vi "Bella_TEA_EnergyMeter_GUI-viremote.vi"() -> (0 "error IO 2":errorcluster)   [LabVIEW 2013]
uses:
  shared programs/GUI_Template/GUI_master/tcp_new_data_event.ctl
  shared programs/GUI_Template/GUI_master/tcp new data cluster.ctl
  VIremote/VIremote.llb/VIremoteFunction.ctl
panel:
  in  "error IO":errorcluster
  in  "Energy Mode::11":enum16{"off", "on"}(ring) caption="Energy Mode"
  in  "triggerlevel::11":dbl=0.5 caption="Trig Level" min=0.0 max=100.0 format="%_4f"
  out "Wavelength::11":i32 caption="Wavelength" min=0 max=5000
  out "tcp data event":T1
  in  "GUIdevice 11":string="BELLA_TEA_PowerMeter"
  in  "insert tag":bool=TRUE
  in  "stop":bool
  out "Reading::11":dbl=0.5 caption="Reading" min=0.0 max=50000.0 format="%_4p"
  # "TEA PLink Energy Meter"
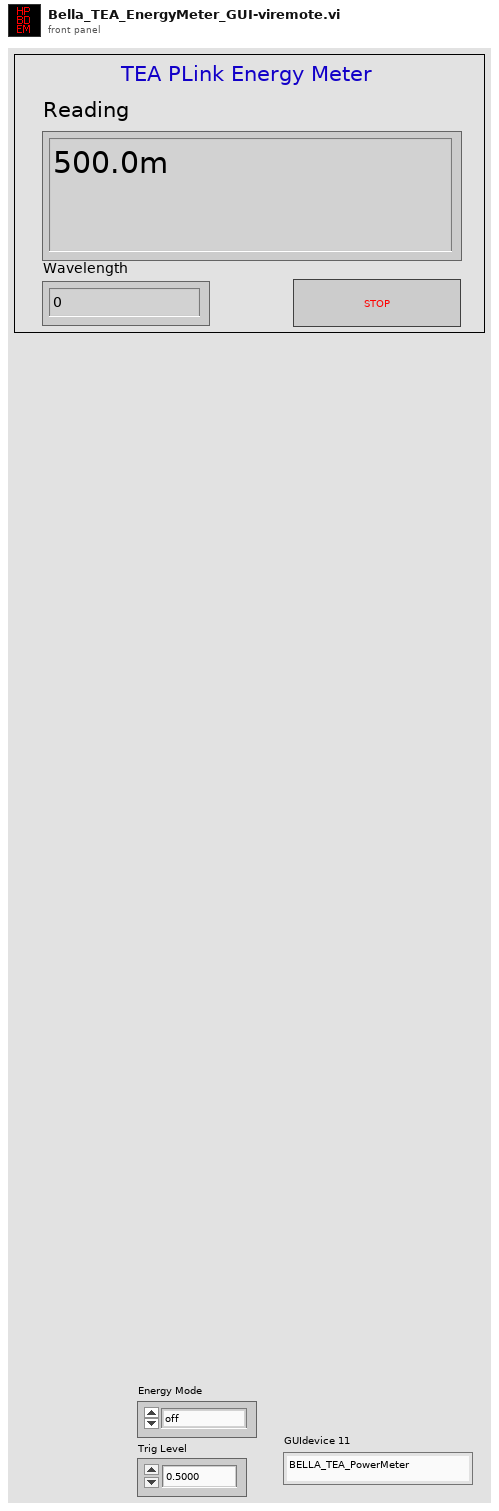
[diagram p1: front panel]
types:
  T1 = typedef "tcp_new_data_event.ctl" = refnum<user-event>
  T2 = typedef "tcp new data cluster.ctl" = cluster{"EventEnum":enum16{"new data", "connection status update"}, "Device name":string}
  T3 = typedef "VIremoteFunction.ctl" = enum16{"Do nothing", "Stop controller", "Close this connection", "Show info panel", "Set VI to control", "Set Accelerometer freq (Hz)", "Show Alert message", "Start Sound Input", "Stop Sound Input", "Set Volume (0-100)", "Set sound output Speaker", "Set sound output Receiver", "Play Sound", "Repeat Sound", "Stop Sound", "Pause Sound", "Resume Sound", "Set panel width of caller (320 or 480)", "Set Panel Size to Portrait", "Set Panel Size to Landscape", "Set Panel Size as Current Orientation", "Allow all UI Orientations", "Send user notification", "Disable Scrolling", "Normal Scrolling", "Page Scrolling", "Set Scroll Offset", "Page Indicator Position"}
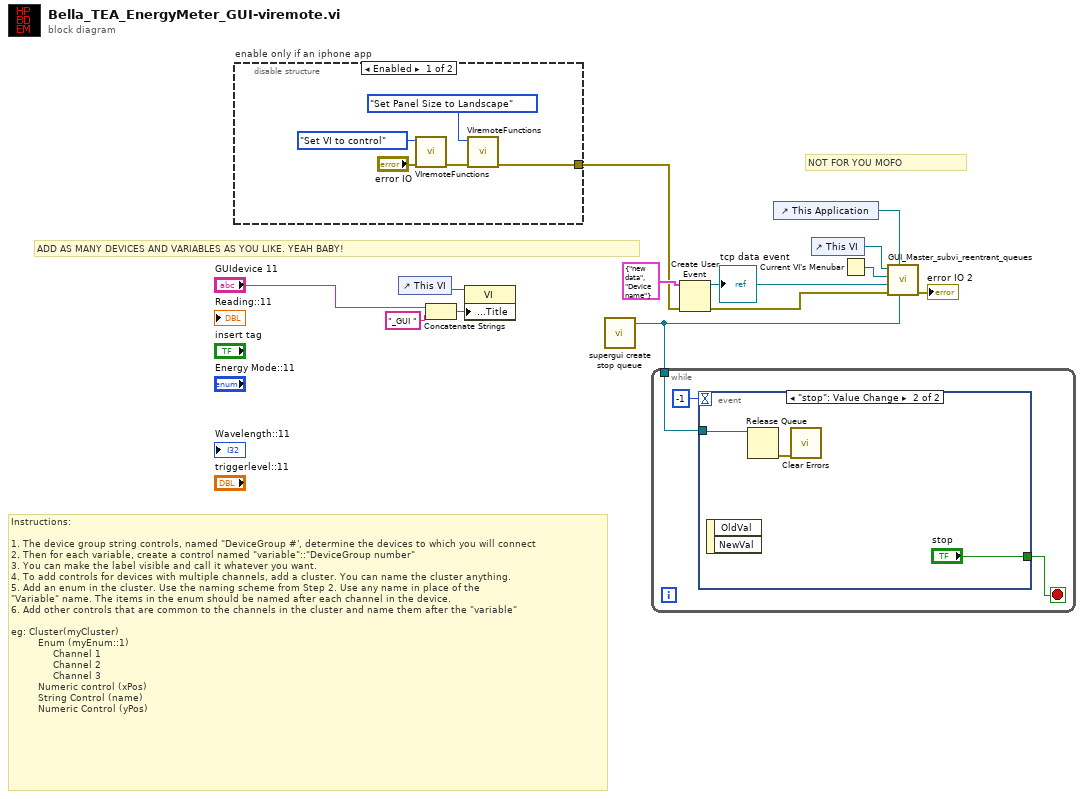
[diagram p0: block diagram]
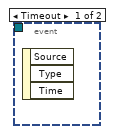
[diagram p2: hidden frame]
diagram:
  # "Instructions:\n\n1. The device group string controls, named \"DeviceGroup #', determine the devices to which you will connect\n2. Then for each variable, create a control named \"variable\"::\"DeviceGroup number\"\n3. You can make the label visible and call it whatever you want.\n4. To add controls for devices with multiple channels, add a cluster. You can name the cluster anything.\n5. Add an enum in the cluster. Use the naming scheme from Step 2. Use any name in place of the \n\"Variable\" name. The items in the enum should be named after each channel in the device. \n6. Add other controls that are common to the channels in the cluster and name them after the \"variable\"\n\neg: Cluster(myCluster)\n         Enum (myEnum::1)\n              Channel 1 \n              Channel 2\n              Channel 3\n         Numeric control (xPos)\n         String Control (name)\n         Numeric Control (yPos)"
  # "ADD AS MANY DEVICES AND VARIABLES AS YOU LIKE. YEAH BABY!"
  # "NOT FOR YOU MOFO"
  n1 = disable-structure "enable only if an iphone app" shown="Enabled" {
    disable-tunnel: [w14 _] -> w7
    frame Enabled {
      n2 = call "VIremoteFunctions.vi"("error in (no error)"="error IO", "Function"=VIremoteFunction."Set VI to control") -> ("error out"=w15:errorcluster)  [unwired: 4 in, 5 out]
      n3 = call "VIremoteFunctions.vi"("error in (no error)"=w15, "Function"=VIremoteFunction."Set Panel Size to Landscape") -> ("error out"=w14:errorcluster)  [unwired: 4 in, 5 out]
    }
    frame Disabled {
    }
  }
  n4 = control-ref of="This VI"() -> (w4:refnum<vi>)
  n5 = Concatenate Strings("GUIdevice 11", "_GUI ") -> (w3:string)
  n6 = property class="VI"(reference=w4, "Front Panel.Title"=w3) -> ()  [unwired: 1 in, 2 out]
  n7 = call "supergui create stop queue.vi"() -> ("STOP Queue out"=w5:refnum<queue>)  [unwired: 11 in]
  n8 = while {
    tunnel: w5 -> [w19]
    stop <- w20 stop-if-true
    n9 = event shown="[1] \"stop\": Value Change" {
      selector: _ -> [_ _]
      dyn-events: _ -> [_ _]
      timeout: -1 -> [_ _]
      tunnel: [_ "stop"] -> w20
      tunnel: w19 -> [_ w22]
      event Timeout {
        n10 = event-data() -> ()  [unwired: 1 in, 3 out]
      }
      event "stop": Value Change {
        n11 = event-data() -> ()  [unwired: 1 in, 2 out]
        n12 = Release Queue(queue=w22) -> (error out=w23:errorcluster)  [unwired: 2 in, 2 out]
        n13 = call <vilib>:"Clear Errors.vi"("error in (no error)"=w23) -> ()  [unwired: 6 in, 1 out]
      }
    }
  }
  n14 = Create User Event(user event datatype=T2 {"EventEnum"=enum."new data", "Device name"="Device name"} ("New Event"), error in=w7) -> (user event=w8:refnum<user-event>, error out=w9:errorcluster)
  "tcp data event" <- w8
  n15 = control-ref of="This Application"() -> (w6:refnum<vi>)
  n16 = control-ref of="This VI"() -> (w12:refnum<vi>)
  n17 = Current VI's Menubar() -> (w11:refnum<k9>)
  n18 = call "GUI_Master_subvi_reentrant_queues.vi"("STOP Queue in"=w5, "This Application"=w6, "error in (no error)"=w9, "tcp data event"=w8, "Caller menu reference"=w11, "Caller VI ref"=w12) -> ("error out"=→"error IO 2":errorcluster)  [unwired: 5 in]
